vi "Configure BERT Pseudo Pattern.vi"(8 "error in (no error)":errorcluster, 10 "Incoming Data Pattern (0: PN9)":i32(ring) items=["PN9", "PN11", "PN15", "PN20", "PN23"], 11 "VISA resource name":refnum<visa-resource-name>) -> (0 "error out":errorcluster, 3 "VISA resource name out":refnum<visa-resource-name>)   [LabVIEW 2018, in "Agilent PSG MXG Series.lvlib"]
doc: "Configures the incoming data pattern for making BER measurements.\n\n<b>Note:</b>\nIt is applicable for N5172B/82B with <b>Option UN7</b> only."
uses:
  Agilent PSG MXG Series.lvlib
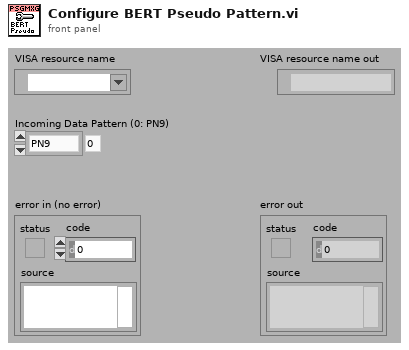
[diagram p1: front panel]
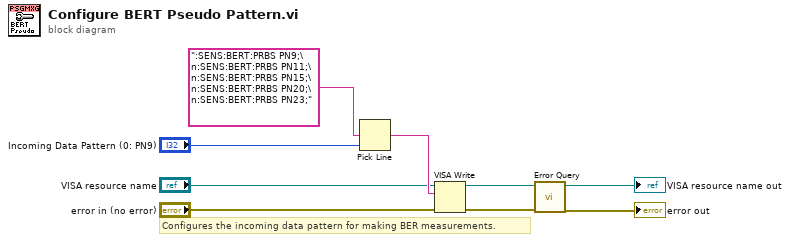
[diagram p0: block diagram]
diagram:
  # "Configures the incoming data pattern for making BER measurements."
  n1 = Pick Line(multi-line string=":SENS:BERT:PRBS PN9;\n:SENS:BERT:PRBS PN11;\n:SENS:BERT:PRBS PN15;\n:SENS:BERT:PRBS PN20;\n:SENS:BERT:PRBS PN23;", line index="Incoming Data Pattern (0: PN9)") -> (output string=w7:string)  [unwired: 1 in]
  n2 = VISA Write(VISA resource name="VISA resource name", write buffer=w7, error in (no error)="error in (no error)") -> (VISA resource name out=w4:refnum<visa-resource-name>, error out=w3:errorcluster)  [unwired: 1 out]
  n3 = call "Error Query.vi"("error in (no error)"=w3, "VISA resource name"=w4) -> ("error out"=→"error out":errorcluster, "VISA resource name out"=→"VISA resource name out":refnum<visa-resource-name>)  [unwired: 6 in, 2 out]
